vi "Hi_Tec_Testing.vi"() -> ()   [LabVIEW 2010]
panel:
  in  "Gas Line Name 4":string="Carrier 1"
  in  "Gas Line Name 3":string="Carrier 2"
  in  "Gas Line Name 2":string="Trace"
  out "Output":dbl format="%.3f"
  in  "Gas Line Name":string="Carrier 1"
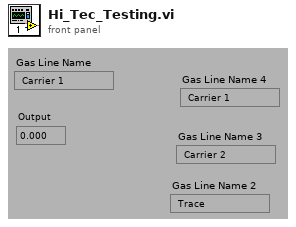
[diagram p1: front panel]
types:
  T1 = enum16{"Q(release) to Volts", "Volts to Q(release)"}
  T2 = typedef "Hi-Tec_calib.ctl" = cluster{"Ref temp (deg C)":dbl, "Ref Pres (mbars)":dbl, "Density at calib conditions":dbl, "Coefficients":dbl[]}
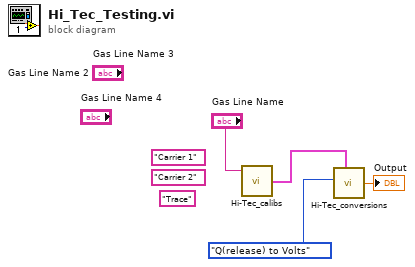
[diagram p0: block diagram]
diagram:
  (unwired) "Trace" ("Gas Line Name")
  (unwired) "Carrier 2" ("Gas Line Name")
  (unwired) "Carrier 1" ("Gas Line Name")
  n1 = call "Hi-Tec_calibs.vi"("Gas Line Name"="Gas Line Name") -> ("Hi-Tec calib"=w4:T2)  [unwired: 3 in, 1 out]
  n2 = call "Hi-Tec_conversions.vi"("Conversion"=T1."Q(release) to Volts", "Hi-Tec calib"=w4) -> ("Output"=→"Output":dbl)  [unwired: 4 in, 1 out]
